vi "Update_RawActPosition.vi"(8 "error in (no error)":errorcluster, 9 "RawActPosition?":dbl, 10 "PV-URL":string, 11 "CS++Motor in":refnum<class "CS++Motor.lvclass">) -> (0 "error out":errorcluster, 3 "CS++Motor out":refnum<class "CS++Motor.lvclass">)   [LabVIEW 2016, in "CS++Motor.lvlib" / "CS++Motor.lvclass"]
doc: "This VI is executed via the corresponding Monitor Actor and delivers the information abot the Raw Act Position of an axis."
uses:
  CS++Motor.lvclass
  CS++Motor.lvclass/CS++Motor.ctl
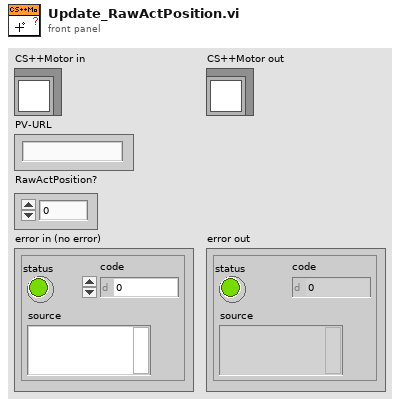
[diagram p1: front panel]
types:
  T1 = cluster{"Update-Msg Name":string, "Update-Msg URLs":string[]}[]
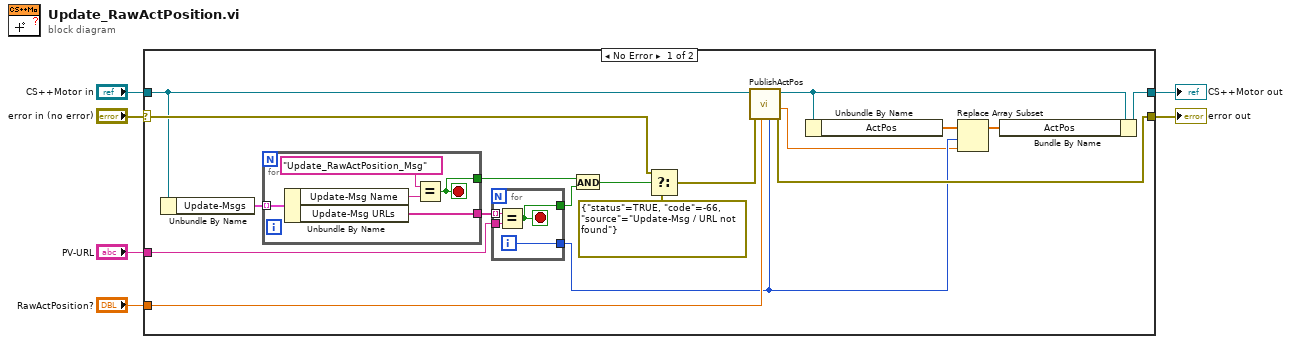
[diagram p0: block diagram]
diagram:
  n1 = case shown="No Error" "error in (no error)" {
    selector: "error in (no error)" -> [w19 w35]
    tunnel: [w10 w35] -> w5
    tunnel: [w14 w34] -> w3
    tunnel: "CS++Motor in" -> [w13 w34]
    tunnel: "RawActPosition?" -> [w9 _]
    tunnel: "PV-URL" -> [w17 _]
    frame No Error {
      n2 = Unbundle By Name(w13) -> ("Update-Msgs"=w20:T1)
      n3 = for {
        tunnel: w20 -> [w33] mode=indexing
        tunnel: [w30] -> w18
        tunnel: [w29] -> w24
        stop <- w29 stop-if-true
        n4 = Unbundle By Name(w33) -> ("Update-Msg Name"=w32:string, "Update-Msg URLs"=w30:string[])
        n5 = Equal?(x="Update_RawActPosition_Msg", y=w32) -> (x = y?=w29:bool)
      }
      n6 = for {
        tunnel: w18 -> [w28] mode=indexing
        tunnel: w17 -> [w27]
        tunnel: [w26] -> w23
        tunnel: [w25] -> w8
        i -> [w25]
        stop <- w26 stop-if-true
        n7 = Equal?(x=w28, y=w27) -> (x = y?=w26:bool)
      }
      n8 = And(x=w24, y=w23) -> (x .and. y?=w22:bool)
      n9 = Select(t=w19, s=w22, f=errorcluster {"status"=TRUE, "code"=-66, "source"="Update-Msg / URL not found"}) -> (s? t:f=w11:errorcluster)
      n10 = call "PublishActPos.vi"("AxisNumber"=w8, "RawActPos"=w9, "error in (no error)"=w11, "CS++Motor in"=w13) -> ("error out"=w10:errorcluster, "ActPos"=w7:dbl, "CS++Motor out"=w12:refnum<class "CS++Motor.lvclass">)  [unwired: 5 in]
      n11 = Unbundle By Name(w12) -> ("ActPos"=w16:dbl[])
      n12 = Replace Array Subset(array=w16, new element=w7, index=w8) -> (w15:dbl[])
      n13 = Bundle By Name(cluster=w12, "ActPos"=w15) -> (w14:refnum<class "CS++Motor.lvclass">)
    }
    frame Error {
    }
  }
  "error out" <- w5
  "CS++Motor out" <- w3
